vi "Channel URL to Channel Meta Data.vi"(1 "Channel URL":string) -> (14 "Channel Name":string, 15 "Channel Type":string, 16 "Channel Number":i32)   [LabVIEW 2015, in "SMI.lvlib" / "Module Detection.lvclass"]
uses:
  Module Detection.lvclass
  <vilib>/regexp/Match Regular Expression.xnode
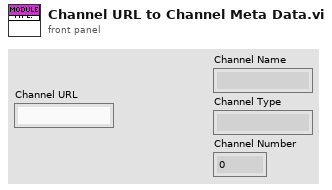
[diagram p1: front panel]
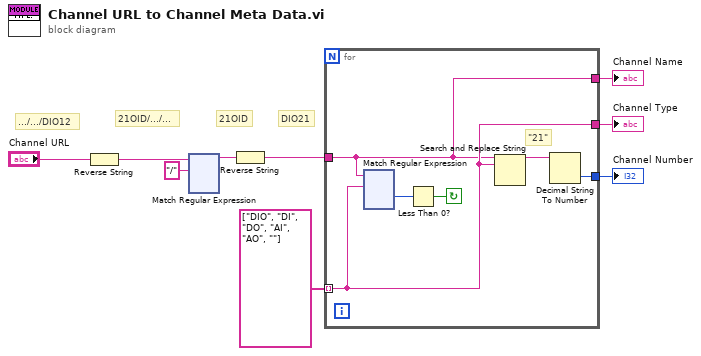
[diagram p0: block diagram]
diagram:
  # ".../.../DIO12"
  # "DIO21"
  # "21OID"
  # "21OID/.../..."
  n1 = Reverse String(1:"Channel URL") -> (0:w5:string)
  n2 = xnode "Match Regular Expression"("input string"=w5, "regular expression"="/") -> ("before match"=w7:string)  [unwired: 4 in, 4 out]
  n3 = Reverse String(1:w7) -> (0:w9:string)
  n4 = for {
    tunnel: string[] ["DIO", "DI", "DO", "AI", "AO", ""] -> [w11] mode=indexing
    tunnel: w9 -> [w10]
    tunnel: [w12] -> w3
    tunnel: [w11] -> w2
    tunnel: [w10] -> w1
    stop <- w14 continue-if-true
    # "\"21\""
    n5 = xnode "Match Regular Expression"("input string"=w10, "regular expression"=w11) -> ("offset past match"=w15:i32)  [unwired: 4 in, 4 out]
    n6 = Less Than 0?(x=w15) -> (x < 0?=w14:bool)
    n7 = Search and Replace String(input string=w10, search string=w11) -> (result string=w13:string)  [unwired: 6 in, 3 out]
    n8 = Decimal String To Number(string=w13) -> (number=w12:i32)  [unwired: 2 in, 1 out]
  }
  "Channel Type" <- w2
  "Channel Number" <- w3
  "Channel Name" <- w1
